vi "High Energy End.vi"() -> ()   [LabVIEW 2016, in "Beamline Sections.lvlib"]
uses:
  Beamline Sections.lvlib
  main/save load/saveload.ctl
panel:
  out "error out":errorcluster
  in  "le fc array output":bool[](array[boolean])
  in  "Tab Control":enum32{"Control", "Readbacks"}(tab)
  out "Analyze magnet readback 2":dbl(graph)=0.8365
  in  "Analyze magnet power supply":dbl(slide)=0.8365 min=0.0 max=1.6 scale=0.0..1.05
  out "He Steerer \nY 2 readback":dbl=2.1859248885760003 format="%#.2g"
  out "He Steerer  X1\nIND":dbl=-2.577066196012 format="%#.2g"
  out "He Steerer Y 1 \nIND":dbl=-0.3914697216320002 format="%#.2g"
  in  "stop":bool
  out "He Quad B readback":dbl=23.541803725959998 format="%#.2g"
  out "He Quad A readback":dbl=12.52186537918 format="%#.2g"
  in  "High Energy Quad A":dbl(knob) scale=17.0..22.0
  in  "High Energy Quad B":dbl(knob) scale=19.0..23.0
  in  "High Energy Y2 steerer":dbl(knob)
  in  "High Energy X steerer":dbl(knob) scale=0.5..3.0
  in  "High Energy Y1 steerer":dbl(knob)
  out "Analyze magnet":bool=TRUE
  out "He  1 and 2Steerer":bool=TRUE
  out "He Quads":bool=TRUE
  in  "Cluster":T1
  out "Analyze magnet object":cluster{string, string, string, string}
  out "Tank exit ion gauge":cluster{string, string, string, string}
  out "Analyze magnet readback":dbl=0.8365
  out "He Steerer X1 Voltage +":dbl=3.6657070700000003
  out "He Steerer X1 Voltage -":dbl=6.334092644
  out "He Steerer Y1 Voltage +":dbl=4.932058047
  out "He Steerer Y1 Voltage -":dbl=5.06749495
  out "He Steerer Y2 Voltage +":dbl=4.216001645
  out "He Steerer Y2 Voltage -":dbl=5.783759862
  out "He Steerer X1 Readback Voltage -":dbl=4.638408521444
  out "He Steerer Y1 Readback  +":dbl=6.277195359484
  out "He Steerer Y1 Readback  -":dbl=3.6955313647279997
  out "He Steerer Y2  Readback +":dbl=4.020661418768
  out "He Steerer Y2  Readback -":dbl=6.050261150048
  out "He Steerer X1 Readback Voltage +":dbl=5.03119189986
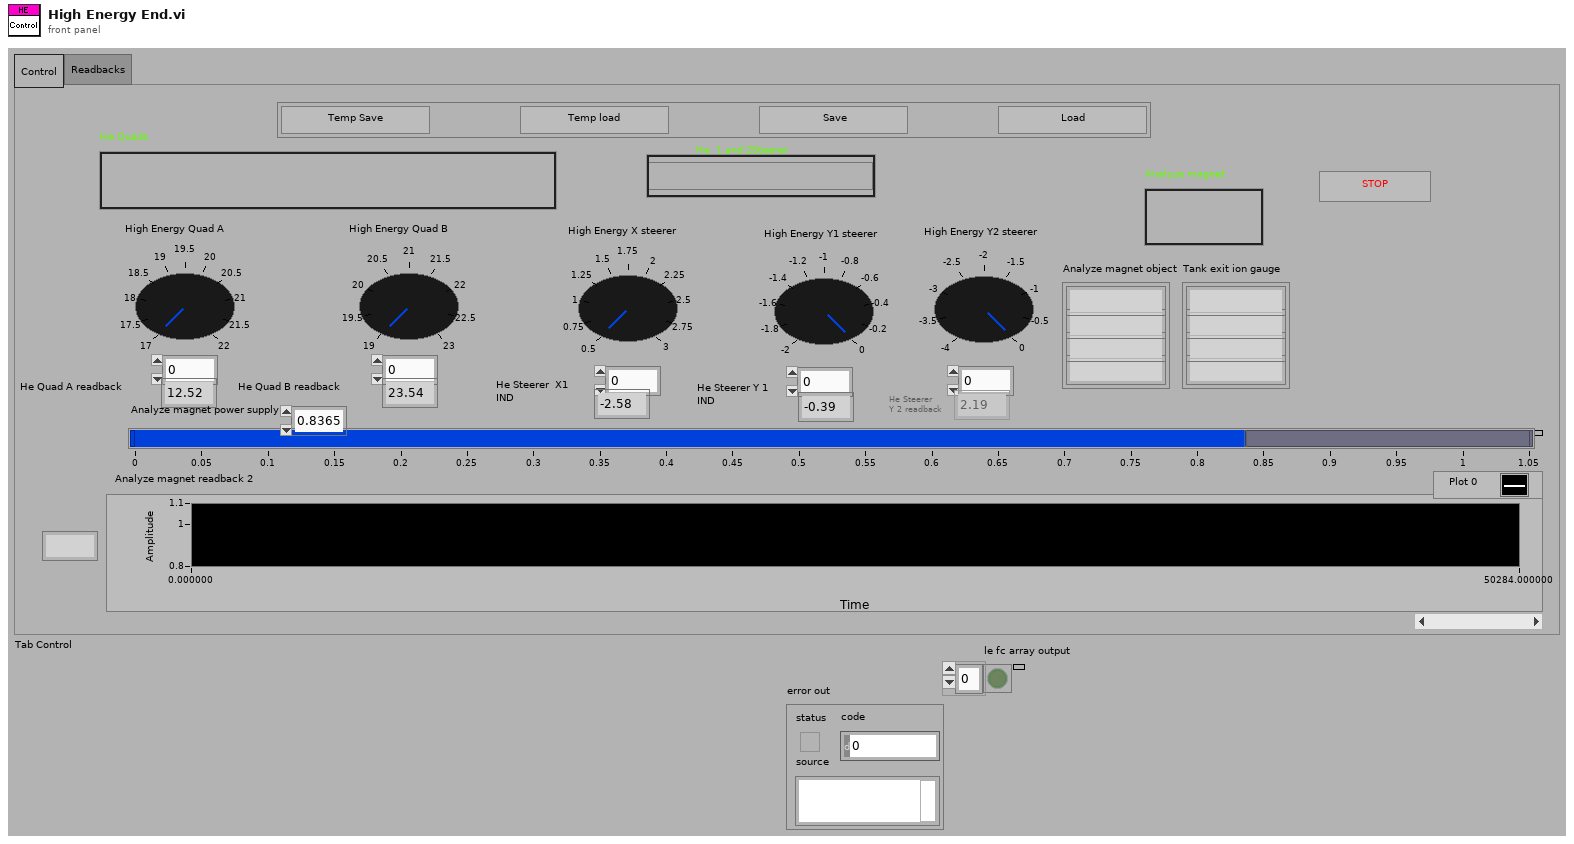
[diagram p1: front panel]
types:
  T1 = typedef "main.lvlib/saveload.ctl" = cluster{"OK Button":bool, "OK Button 2":bool, "OK Button 3":bool, "OK Button 4":bool}
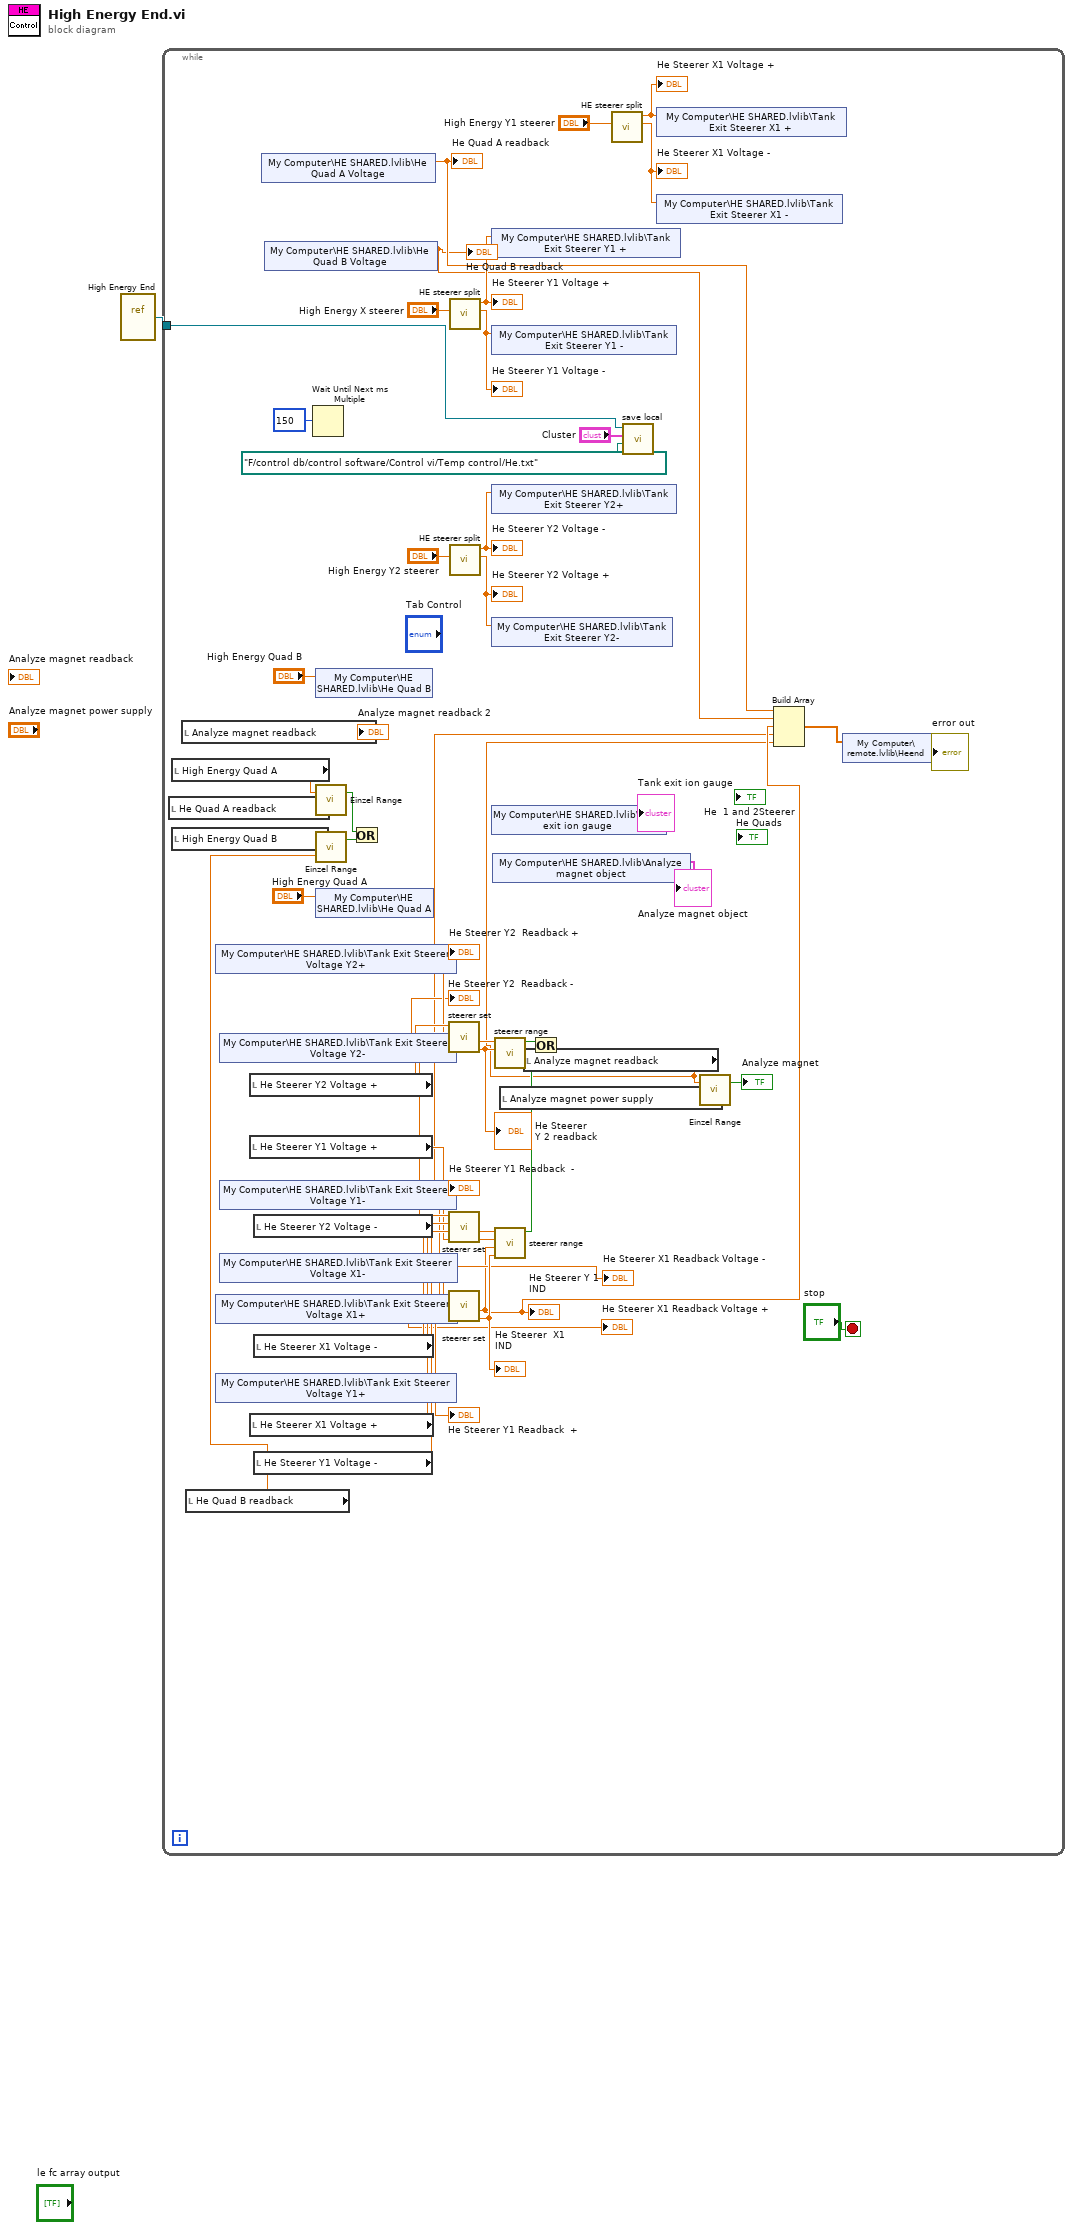
[diagram p0: block diagram]
diagram:
  n1 = vi-ref "High Energy End.vi"() -> (w1:refnum<vi>)
  n2 = while {
    tunnel: w1 -> [w25]
    stop <- "stop" stop-if-true
    n3 = local read "He Quad A readback"() -> (w51:dbl)
    n4 = local read "High Energy Quad A"() -> (w52:dbl)
    n5 = local read "High Energy Quad B"() -> (w50:dbl)
    n6 = local read "Analyze magnet readback"() -> (→"Analyze magnet readback 2":dbl)
    n7 = local read "He Quad B readback"() -> (w49:dbl)
    n8 = shared-variable "My Computer\\HE SHARED.lvlib\\Tank Exit Steerer Voltage Y2+"() -> (w14:dbl)  [unwired: 1 in, 1 out]
    "He Steerer Y2  Readback +" <- w14
    n9 = shared-variable "My Computer\\HE SHARED.lvlib\\Tank Exit Steerer Voltage X1+"() -> (w12:dbl)  [unwired: 1 in, 1 out]
    "He Steerer X1 Readback Voltage +" <- w12
    n10 = shared-variable "My Computer\\HE SHARED.lvlib\\Tank Exit Steerer Voltage Y1+"() -> (w15:dbl)  [unwired: 1 in, 1 out]
    "He Steerer Y1 Readback  +" <- w15
    n11 = shared-variable "My Computer\\HE SHARED.lvlib\\Tank Exit Steerer Voltage Y2-"() -> (w13:dbl)  [unwired: 1 in, 1 out]
    "He Steerer Y2  Readback -" <- w13
    n12 = shared-variable "My Computer\\HE SHARED.lvlib\\Tank Exit Steerer Voltage Y1-"() -> (w5:dbl)  [unwired: 1 in, 1 out]
    "He Steerer Y1 Readback  -" <- w5
    n13 = shared-variable "My Computer\\HE SHARED.lvlib\\Tank Exit Steerer Voltage X1-"() -> (w11:dbl)  [unwired: 1 in, 1 out]
    "He Steerer X1 Readback Voltage -" <- w11
    n14 = local read "He Steerer Y2 Voltage +"() -> (w40:dbl)
    n15 = local read "He Steerer Y1 Voltage +"() -> (w43:dbl)
    n16 = local read "He Steerer X1 Voltage +"() -> (w45:dbl)
    n17 = local read "He Steerer Y2 Voltage -"() -> (w39:dbl)
    n18 = local read "He Steerer X1 Voltage -"() -> (w46:dbl)
    n19 = local read "He Steerer Y1 Voltage -"() -> (w44:dbl)
    n20 = shared-variable "My Computer\\HE SHARED.lvlib\\He Quad A Voltage"() -> (w8:dbl)  [unwired: 1 in, 1 out]
    "He Quad A readback" <- w8
    n21 = shared-variable "My Computer\\HE SHARED.lvlib\\He Quad B Voltage"() -> (w7:dbl)  [unwired: 1 in, 1 out]
    "He Quad B readback" <- w7
    n22 = Wait Until Next ms Multiple(millisecond multiple=u32 150) -> ()  [unwired: 1 out]
    n23 = shared-variable "My Computer\\HE SHARED.lvlib\\He Quad B"("High Energy Quad B") -> ()  [unwired: 1 in, 1 out]
    n24 = call "Einzel Range.vi"("Inj image Readback"=w51, "Inj image Einzel Set"=w52) -> ("Einzel  Range"=w48:bool)  [unwired: 1 out]
    n25 = call "Einzel Range.vi"("Inj image Readback"=w49, "Inj image Einzel Set"=w50) -> ("Einzel  Range"=w47:bool)  [unwired: 1 out]
    n26 = shared-variable "My Computer\\HE SHARED.lvlib\\He Quad A"("High Energy Quad A") -> ()  [unwired: 1 in, 1 out]
    n27 = Or(x=w48, y=w47) -> ()  [unwired: 1 out]
    n28 = call "steerer set.vi"("Injector image X  -"=w40, "Injector image X +"=w39, "Injector image Y  -"=w13, "Injector image Y +"=w14) -> ("Steerer X"=w37:dbl, "Steerer Y"=w38:dbl)  [unwired: 4 out]
    "He Steerer \nY 2 readback" <- w38
    n29 = call "steerer set.vi"("Injector image X  -"=w46, "Injector image X +"=w45, "Injector image Y  -"=w44, "Injector image Y +"=w43) -> ("Steerer X"=w42:dbl, "Steerer Y"=w41:dbl)  [unwired: 4 out]
    n30 = call "steerer set.vi"("Injector image X  -"=w11, "Injector image X +"=w12, "Injector image Y  -"=w5, "Injector image Y +"=w15) -> ("Steerer X"=w6:dbl, "Steerer Y"=w24:dbl)  [unwired: 4 out]
    "He Steerer Y 1 \nIND" <- w6
    "He Steerer  X1\nIND" <- w24
    n31 = call "HE steerer split.vi"("Steerer in"="High Energy X steerer") -> ("Steerer +"=w21:dbl, "Steerer -"=w20:dbl)  [unwired: 7 out]
    "He Steerer Y1 Voltage +" <- w21
    "He Steerer Y1 Voltage -" <- w20
    n32 = call "HE steerer split.vi"("Steerer in"="High Energy Y2 steerer") -> ("Steerer +"=w17:dbl, "Steerer -"=w16:dbl)  [unwired: 7 out]
    "He Steerer Y2 Voltage +" <- w16
    "He Steerer Y2 Voltage -" <- w17
    n33 = shared-variable "My Computer\\HE SHARED.lvlib\\Tank Exit Steerer Y1 +"(w21) -> ()  [unwired: 1 in, 1 out]
    n34 = shared-variable "My Computer\\HE SHARED.lvlib\\Tank Exit Steerer Y1 -"(w20) -> ()  [unwired: 1 in, 1 out]
    n35 = shared-variable "My Computer\\HE SHARED.lvlib\\Tank Exit Steerer Y2+"(w17) -> ()  [unwired: 1 in, 1 out]
    n36 = shared-variable "My Computer\\HE SHARED.lvlib\\Tank Exit Steerer Y2-"(w16) -> ()  [unwired: 1 in, 1 out]
    n37 = shared-variable "My Computer\\HE SHARED.lvlib\\Tank exit ion gauge"() -> (→"Tank exit ion gauge":cluster{string, string, string, string})  [unwired: 1 in, 1 out]
    n38 = shared-variable "My Computer\\HE SHARED.lvlib\\Analyze magnet object"() -> (→"Analyze magnet object":cluster{string, string, string, string})  [unwired: 1 in, 1 out]
    n39 = call "steerer range.vi"("Steerer Set Y"=w38, "Steerer X Set"=w37) -> ("Steerer within range"=w35:bool)  [unwired: 5 in]
    n40 = call "steerer range.vi"("Steerer Y Voltage"=w24, "Steerer X Voltage"=w6, "Steerer Set Y"=w41, "Steerer X Set"=w42) -> ("Steerer within range"=w36:bool)  [unwired: 3 in]
    n41 = local read "Analyze magnet power supply"() -> (w34:dbl)
    n42 = local read "Analyze magnet readback"() -> (w4:dbl)
    n43 = Or(x=w35, y=w36) -> ()  [unwired: 1 out]
    n44 = call "HE steerer split.vi"("Steerer in"="High Energy Y1 steerer") -> ("Steerer +"=w18:dbl, "Steerer -"=w19:dbl)  [unwired: 7 out]
    "He Steerer X1 Voltage +" <- w18
    "He Steerer X1 Voltage -" <- w19
    n45 = call "save local.vi"("file path (use dialog)"=path "F:/control db/control software/Control vi/Temp control/He.txt", "Ring"="Cluster", "VI Refnum"=w25) -> ()  [unwired: 2 out]
    n46 = shared-variable "My Computer\\HE SHARED.lvlib\\Tank Exit Steerer X1 +"(w18) -> ()  [unwired: 1 in, 1 out]
    n47 = shared-variable "My Computer\\HE SHARED.lvlib\\Tank Exit Steerer X1 -"(w19) -> ()  [unwired: 1 in, 1 out]
    n48 = call "Einzel Range.vi"("Inj image Readback"=w34, "Inj image Einzel Set"=w4) -> ("Einzel  Range"=→"Analyze magnet":bool)  [unwired: 1 out]
    n49 = Build Array(w8, w7, w6, w5, w4) -> (w3:dbl[])
    n50 = shared-variable "My Computer\\remote.lvlib\\Heend"(w3) -> (error out=→"error out":errorcluster)  [unwired: 1 in]
  }
